vi "Create Command.vi"(10 "Save Path":path) -> (3 "Save.lvclass":refnum<class "Save.lvclass">)   [LabVIEW 2010, in "Save.lvclass"]
doc: "This instance of Create Command.vi writes the value of Save Path to the data stored within Save.lvclass."
uses:
  Save.lvclass
  Save.lvclass/Save.ctl
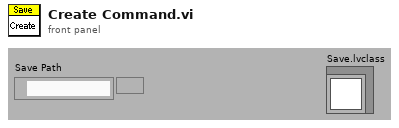
[diagram p1: front panel]
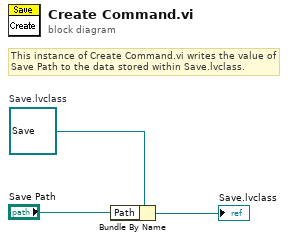
[diagram p0: block diagram]
diagram:
  w3 = refnum<class "Save.lvclass"> refnum  # Save.lvclass
  # "This instance of Create Command.vi writes the value of Save Path to the data stored within Save.lvclass."
  n1 = Bundle By Name "Bundle By Name"(cluster=w3, "Path"="Save Path") -> (→"Save.lvclass":refnum<class "Save.lvclass">)
